vi "ObtainPublicQueues.vi"(8 "error in (no error)":errorcluster, 10 "Min Queue Buffer":i32=10, 11 "DAQmx":refnum<class "DAQmx.lvclass">) -> (0 "error out":errorcluster, 3 "DAQmx out":refnum<class "DAQmx.lvclass">)   [LabVIEW 2019, in "DAQmx.lvclass"]
uses:
  DAQmx.lvclass
  DAQmx.lvclass/DAQmx.ctl
panel:
  # "For instructions on how to use the JKI State Machine Objects, examples and video tutorials, visit:\nhttp://jki.net/state-machine-objects/\n\nJKI State Machine Objects™\nhttp://jki.net/state-machine-objects/\nCopyright (C) 2005-2015, JKI <info@jki.net>\nALL RIGHTS RESERVED"
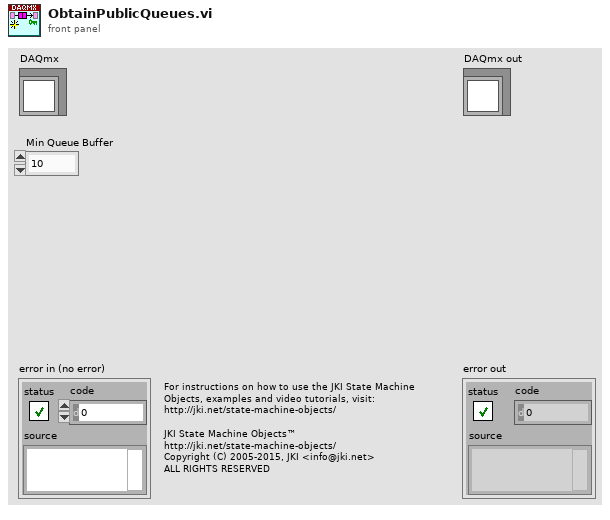
[diagram p1: front panel]
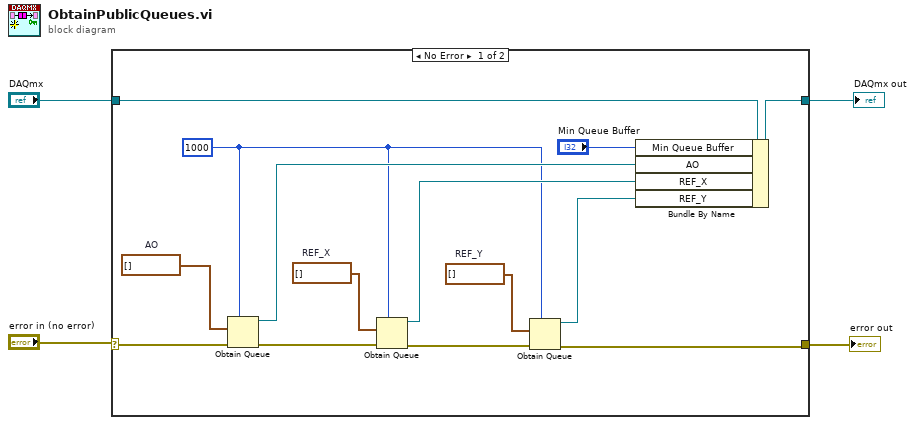
[diagram p0: block diagram]
diagram:
  n1 = case shown="No Error" "error in (no error)" {
    selector: "error in (no error)" -> [w16 w20]
    tunnel: [w8 w20] -> w2
    tunnel: [w17 w19] -> w3
    tunnel: "DAQmx" -> [w18 w19]
    frame No Error {
      w6 = 1000 ("Queue Buffer")
      w13 = waveform(dbl)[] []  # REF_Y
      w14 = waveform(dbl)[] []  # REF_X
      w15 = waveform(dbl)[] []  # AO
      n2 = Obtain Queue(max queue size (-1, unlimited)=w6, element data type=w15, error in (no error)=w16) -> (queue out=w7:refnum<queue>, error out=w10:errorcluster)  [unwired: 2 in, 1 out]
      n3 = Obtain Queue(max queue size (-1, unlimited)=w6, element data type=w14, error in (no error)=w10) -> (queue out=w12:refnum<queue>, error out=w9:errorcluster)  [unwired: 2 in, 1 out]
      n4 = Obtain Queue(max queue size (-1, unlimited)=w6, element data type=w13, error in (no error)=w9) -> (queue out=w11:refnum<queue>, error out=w8:errorcluster)  [unwired: 2 in, 1 out]
      n5 = Bundle By Name(cluster=w18, "Min Queue Buffer"="Min Queue Buffer", "AO"=w7, "REF_X"=w12, "REF_Y"=w11) -> (w17:refnum<class "DAQmx.lvclass">)
    }
    frame Error {
    }
  }
  "error out" <- w2
  "DAQmx out" <- w3
